vi "4155C Transfer-FPP Config SMUs.vi"(0 "VISA resource name in":refnum<visa-resource-name>, 1 "sweep method":u16(ring) items=["Continuous", "Pulsed"], 2 "Gate mode":u16(ring) items=["Auto", "Limited", "Fixed"], 3 "Gate Range":u8(slide)=6 max=11 scale=0.0..11.0, 5 "Pulse period":dbl=0.005 min=0.005 max=1.0 step=0.0001 format="%.4f", 7 "Pulse width":dbl=0.0005 min=0.0005 max=0.1 step=0.0001 format="%.4f", 9 "Base voltage":dbl format="%^.4e", 11 "error in (no error)":errorcluster, 13 "Source/drain mode":u16(ring) items=["Auto", "Limited", "Fixed"], 14 "Source/drain Range":u8(slide)=6 max=11 scale=0.0..11.0) -> (4 "VISA Resource Name out":refnum<visa-resource-name>, 15 "error out":errorcluster)   [LabVIEW 2016]
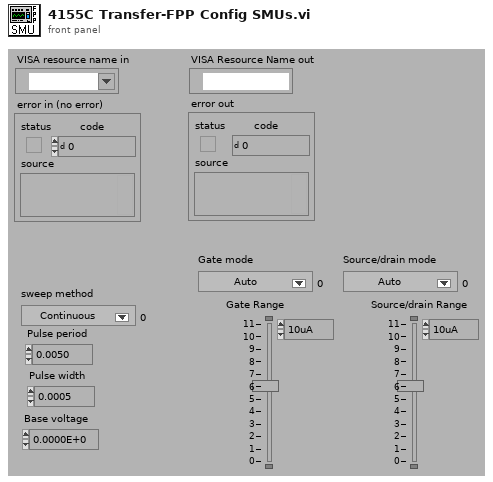
[diagram p1: front panel]
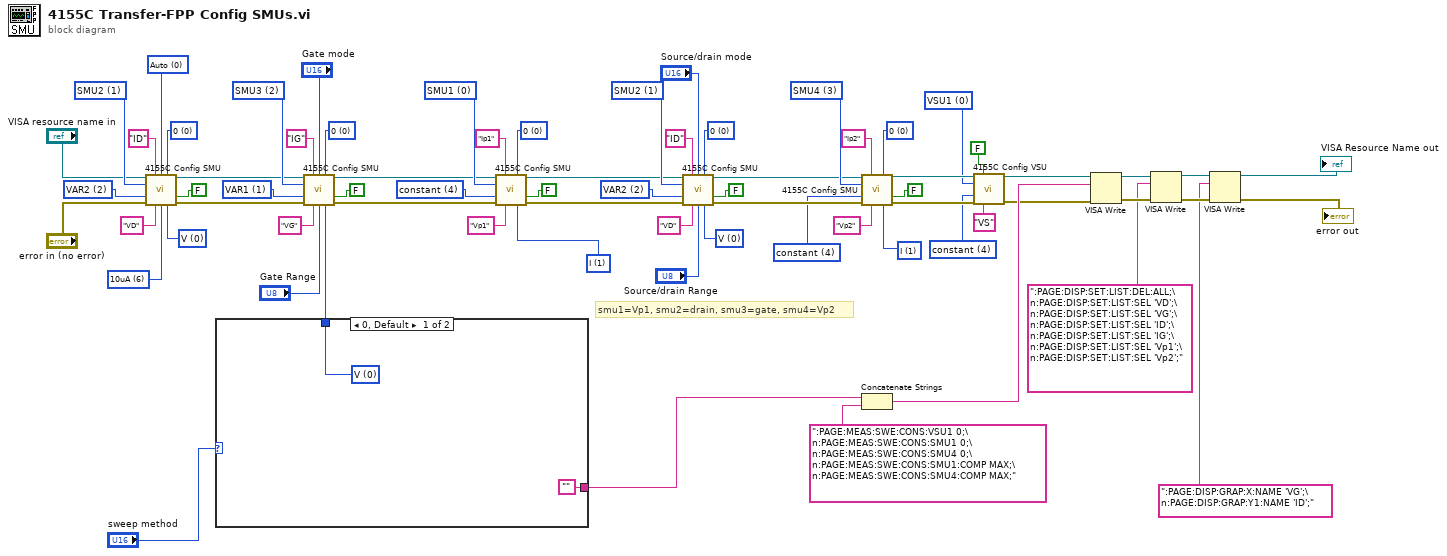
[diagram p0: block diagram]
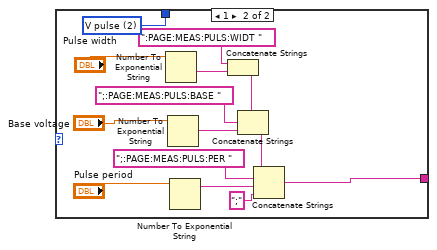
[diagram p2: hidden frame]
diagram:
  w14 = u32 4 items=["disabled  ", "VAR1  ", "VAR2  ", "VAR1'  ", "constant  "] ("function")
  w15 = u32 0 items=["VSU1  ", "VSU2  "] ("unit to configure")
  w21 = u32 4 items=["disabled  ", "VAR1  ", "VAR2  ", "VAR1'  ", "constant  "] ("function")
  w25 = u32 1 items=["V  ", "I  ", "V pulse  ", "I pulse  ", "  common  "] ("mode")
  w26 = u16 0 items=["Auto", "Limited", "Fixed"] ("Range mode")
  w27 = u8 6 items=["10fA  ", "100fA  ", "1nA  ", "10nA", "100nA", "1uA", "10uA", "100uA", "1mA", "10mA", "100mA", "1A"] ("Range")
  w32 = u32 1 items=["SMU1  ", "SMU2  ", "SMU3  ", "SMU4  ", "SMU5  ", "SMU6  "] ("unit to configure")
  w33 = u32 2 items=["disabled  ", "VAR1  ", "VAR2  ", "VAR1'  ", "constant  "] ("function")
  w35 = u32 0 items=["0  ", "10K Ohms  ", "100K Ohms  ", "1M Ohms  "] ("series resistance *")
  w36 = u32 0 items=["V  ", "I  ", "V pulse  ", "I pulse  ", "  common  "] ("mode")
  w50 = u32 0 items=["0  ", "10K Ohms  ", "100K Ohms  ", "1M Ohms  "] ("series resistance *")
  w52 = u32 3 items=["SMU1  ", "SMU2  ", "SMU3  ", "SMU4  ", "SMU5  ", "SMU6  "] ("unit to configure")
  w55 = u32 0 items=["V  ", "I  ", "V pulse  ", "I pulse  ", "  common  "] ("mode")
  w56 = u32 0 items=["0  ", "10K Ohms  ", "100K Ohms  ", "1M Ohms  "] ("series resistance *")
  w58 = u32 2 items=["disabled  ", "VAR1  ", "VAR2  ", "VAR1'  ", "constant  "] ("function")
  w59 = u32 1 items=["SMU1  ", "SMU2  ", "SMU3  ", "SMU4  ", "SMU5  ", "SMU6  "] ("unit to configure")
  w62 = u32 0 items=["0  ", "10K Ohms  ", "100K Ohms  ", "1M Ohms  "] ("series resistance *")
  w64 = u32 4 items=["disabled  ", "VAR1  ", "VAR2  ", "VAR1'  ", "constant  "] ("function")
  w65 = u32 0 items=["SMU1  ", "SMU2  ", "SMU3  ", "SMU4  ", "SMU5  ", "SMU6  "] ("unit to configure")
  w40 = u32 1 items=["V  ", "I  ", "V pulse  ", "I pulse  ", "  common  "] ("mode")
  w68 = u32 0 items=["0  ", "10K Ohms  ", "100K Ohms  ", "1M Ohms  "] ("series resistance *")
  w70 = u32 1 items=["disabled  ", "VAR1  ", "VAR2  ", "VAR1'  ", "constant  "] ("function")
  w71 = u32 2 items=["SMU1  ", "SMU2  ", "SMU3  ", "SMU4  ", "SMU5  ", "SMU6  "] ("unit to configure")
  # "smu1=Vp1, smu2=drain, smu3=gate, smu4=Vp2"
  n1 = call "4155C Config SMU.vi"("VISA session"="VISA resource name in", "I name (max 6 chars)"="ID", "Range mode"=w26, "series resistance *"=w35, "unit to configure"=w32, "function"=w33, "standby"=FALSE, "error in (no error)"="error in (no error)", "V name (max 6 chars)"="VD", "Range"=w27, "mode"=w36) -> ("dup VISA resource name"=w29:refnum<visa-resource-name>, "error out"=w30:errorcluster)  [unwired: 3 in]
  n2 = case shown="0, Default" "sweep method" {
    tunnel: [w73 w87] -> w39
    tunnel: ["" w78] -> w24
    frame 0, Default {
      w73 = u32 0 items=["V  ", "I  ", "V pulse  ", "I pulse  ", "  common  "] ("mode")
    }
    frame 1 {
      w87 = u32 2 items=["V  ", "I  ", "V pulse  ", "I pulse  ", "  common  "] ("mode")
      n3 = Number To Exponential String(number="Pulse width") -> (E-format string=w86:string)  [unwired: 3 in]
      n4 = Number To Exponential String(number="Base voltage") -> (E-format string=w82:string)  [unwired: 3 in]
      n5 = Number To Exponential String(number="Pulse period") -> (E-format string=w79:string)  [unwired: 3 in]
      n6 = Concatenate Strings(":PAGE:MEAS:PULS:WIDT " ("Substring"), w86) -> (w84:string)
      n7 = Concatenate Strings(w84, ";:PAGE:MEAS:PULS:BASE " ("Substring"), w82) -> (w80:string)
      n8 = Concatenate Strings(w80, ";:PAGE:MEAS:PULS:PER " ("Substring"), w79, ";" ("Substring")) -> (w78:string)
    }
  }
  n9 = call "4155C Config SMU.vi"("VISA session"=w29, "I name (max 6 chars)"="IG", "Range mode"="Gate mode", "series resistance *"=w68, "unit to configure"=w71, "function"=w70, "standby"=FALSE, "error in (no error)"=w30, "V name (max 6 chars)"="VG", "Range"="Gate Range", "mode"=w39) -> ("dup VISA resource name"=w47:refnum<visa-resource-name>, "error out"=w46:errorcluster)  [unwired: 3 in]
  n10 = call "4155C Config SMU.vi"("VISA session"=w47, "I name (max 6 chars)"="Ip1", "series resistance *"=w62, "unit to configure"=w65, "function"=w64, "standby"=FALSE, "error in (no error)"=w46, "V name (max 6 chars)"="Vp1", "mode"=w40) -> ("dup VISA resource name"=w44:refnum<visa-resource-name>, "error out"=w45:errorcluster)  [unwired: 5 in]
  n11 = call "4155C Config SMU.vi"("VISA session"=w44, "I name (max 6 chars)"="ID", "Range mode"="Source/drain mode", "series resistance *"=w56, "unit to configure"=w59, "function"=w58, "standby"=FALSE, "error in (no error)"=w45, "V name (max 6 chars)"="VD", "Range"="Source/drain Range", "mode"=w55) -> ("dup VISA resource name"=w43:refnum<visa-resource-name>, "error out"=w42:errorcluster)  [unwired: 3 in]
  n12 = call "4155C Config SMU.vi"("VISA session"=w43, "I name (max 6 chars)"="Ip2", "series resistance *"=w50, "unit to configure"=w52, "function"=w21, "standby"=FALSE, "error in (no error)"=w42, "V name (max 6 chars)"="Vp2", "mode"=w25) -> ("dup VISA resource name"=w19:refnum<visa-resource-name>, "error out"=w20:errorcluster)  [unwired: 5 in]
  n13 = Concatenate Strings(w24, ":PAGE:MEAS:SWE:CONS:VSU1 0;\n:PAGE:MEAS:SWE:CONS:SMU1 0;\n:PAGE:MEAS:SWE:CONS:SMU4 0;\n:PAGE:MEAS:SWE:CONS:SMU1:COMP MAX;\n:PAGE:MEAS:SWE:CONS:SMU4:COMP MAX;" ("write buffer (\"\")")) -> (w22:string)
  n14 = call "4155C Config VSU.vi"("VISA session"=w19, "standby"=FALSE, "unit to configure"=w15, "function"=w14, "error in (no error)"=w20, "V name (max 6 chars)"="VS") -> ("dup VISA resource name"=w17:refnum<visa-resource-name>, "error out"=w18:errorcluster)  [unwired: 8 in]
  n15 = VISA Write(VISA resource name=w17, write buffer=w22, error in (no error)=w18) -> (VISA resource name out=w8:refnum<visa-resource-name>, error out=w3:errorcluster)  [unwired: 1 out]
  n16 = VISA Write(VISA resource name=w8, write buffer=":PAGE:DISP:SET:LIST:DEL:ALL;\n:PAGE:DISP:SET:LIST:SEL 'VD';\n:PAGE:DISP:SET:LIST:SEL 'VG';\n:PAGE:DISP:SET:LIST:SEL 'ID';\n:PAGE:DISP:SET:LIST:SEL 'IG';\n:PAGE:DISP:SET:LIST:SEL 'Vp1';\n:PAGE:DISP:SET:LIST:SEL 'Vp2';" ("write buffer (\"\")"), error in (no error)=w3) -> (VISA resource name out=w7:refnum<visa-resource-name>, error out=w4:errorcluster)  [unwired: 1 out]
  n17 = VISA Write(VISA resource name=w7, write buffer=":PAGE:DISP:GRAP:X:NAME 'VG';\n:PAGE:DISP:GRAP:Y1:NAME 'ID';" ("write buffer (\"\")"), error in (no error)=w4) -> (VISA resource name out=→"VISA Resource Name out":refnum<visa-resource-name>, error out=→"error out":errorcluster)  [unwired: 1 out]
